vi "On Failure.vi"(8 "error in (no error)":errorcluster, 9 "Session In":refnum<class "Session.lvclass">, 11 "SOL Auth in":refnum<class "SOL Auth.lvclass">) -> (0 "error out":errorcluster, 1 "Session":refnum<class "Session.lvclass">, 2 "Response":refnum<class "Response.lvclass">, 3 "SOL Auth out":refnum<class "SOL Auth.lvclass">)   [LabVIEW 2020, in "Summer of LabVIEW.lvlib" / "SOL Auth.lvclass"]
uses:
  SOL Auth.lvclass
  <vilib>/IlluminatedG/IG HTTP Utils/HTTP Utils/Response/Response.lvclass
  <vilib>/IlluminatedG/IG HTTP Server/HTTP Server/Session/Session.lvclass
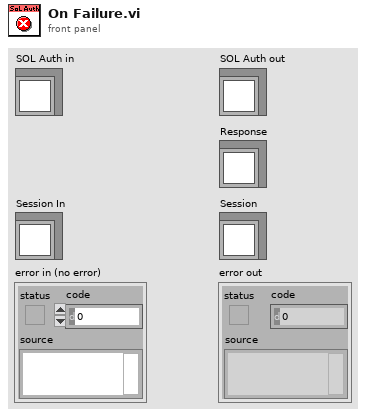
[diagram p1: front panel]
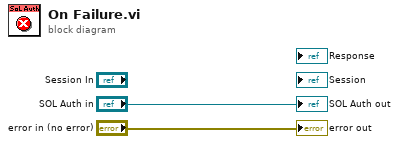
[diagram p0: block diagram]
diagram:
  "error out" <- "error in (no error)"
  "SOL Auth out" <- "SOL Auth in"
